vi "Host Image Acquisition Loop.vi"(8 "error in":errorcluster) -> (0 "error out":errorcluster)   [LabVIEW 2013]
doc: "Loop handles the image acquisition communication to FPGA.\nInitialize - Queues up the intialize states\n\nExit"
uses:
  Host Image Acquisition Module Enum.ctl
  Message Passing/MsgQ Loops enum.ctl
  System Status/Status FG Enum.ctl
  File IO/Save Image Module Enum.ctl
  Image Acquisition Settings FG Enum.ctl
  Globals/Simulation Settings Global.vi
  Common/State Machines/State Machine Lib.lvlib
  Message Passing/Main MsgQ.lvlib
panel:
  out "State":string
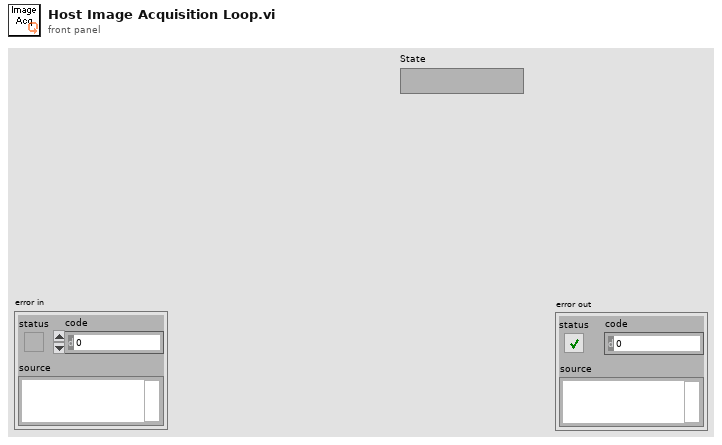
[diagram p1: front panel]
types:
  T1 = typedef "State Machine Lib.lvlib/STATE cluster.ctl" = cluster{"State":string, "Parameters":variant}
  T2 = typedef "Host Image Acquisition Module Enum.ctl" = enum16{"Open FPGA", "Initialize DMA FIFO", "Load Sim Images", "Initialize Acquisition", "Update Sector Parameters", "Start Acquisition", "Aquire Image", "Read Averages", "Cancel Acquisition", "Close FPGA"}
  T3 = typedef "Main MsgQ.lvlib/MsgQ Loops enum.ctl" = enum16{"User Interface", "Image Acq"}
  T4 = typedef "Status FG Enum.ctl" = enum16{"Reset", "Read", "Write"}
  T5 = typedef "Save Image Module Enum.ctl" = enum16{"Create File", "Write to File", "Status", "Close File"}
  T6 = typedef "Image Acquisition Settings FG Enum.ctl" = enum16{"Read", "Write"}
  T7 = typedef "Simulation Settings Cluster.ctl" = cluster{"Sim Enabled?":bool, "Sim Path":path}
  T8 = typedef "Acquisition Settings Cluster.ctl" = cluster{"Image Width":u32, "Image Height":u32, "Frames To Acquire":u32, "Signal Mapping":enum8{"Standard", "Basler 10-tap", "Vosskühler 10-tap"}, "DMA Buffer Size\n(In Images)":u32}
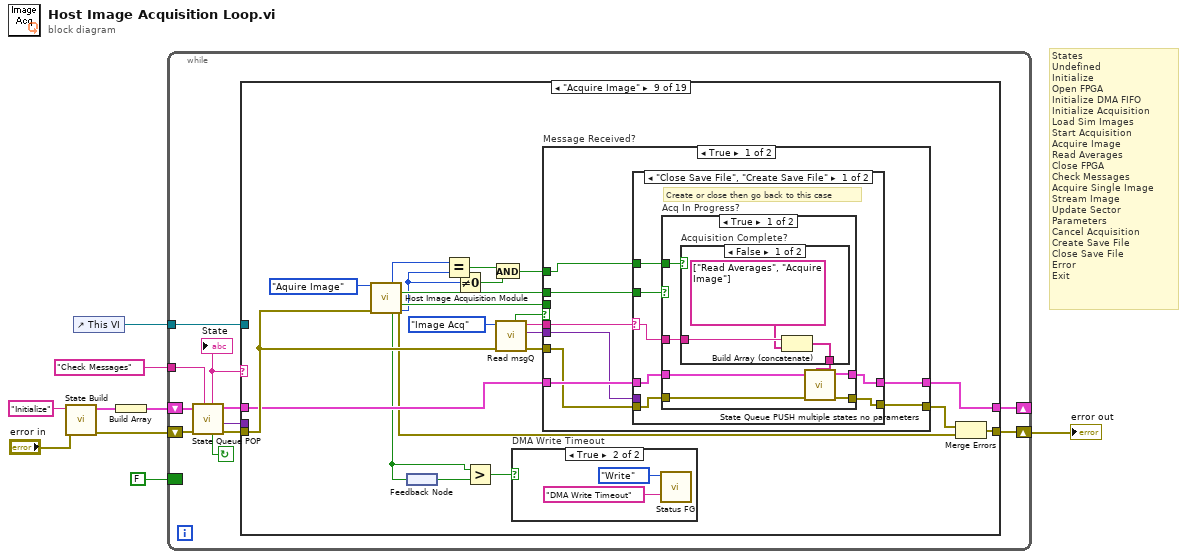
[diagram p0: block diagram]
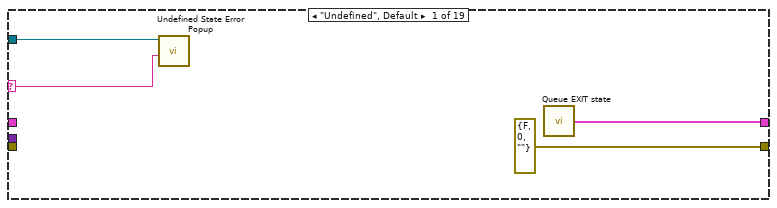
[diagram p2: hidden frame]
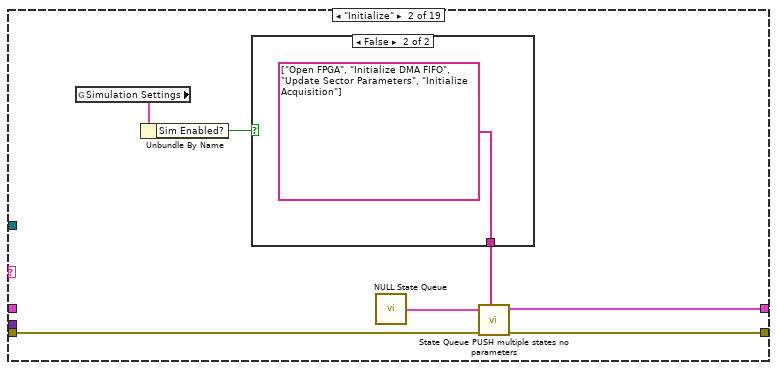
[diagram p3: hidden frame]
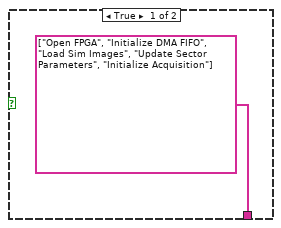
[diagram p4: hidden frame]
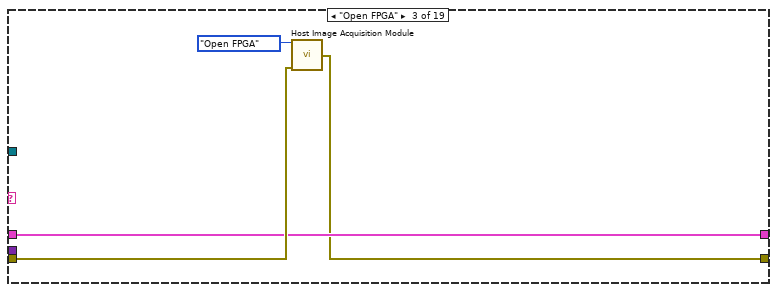
[diagram p5: hidden frame]
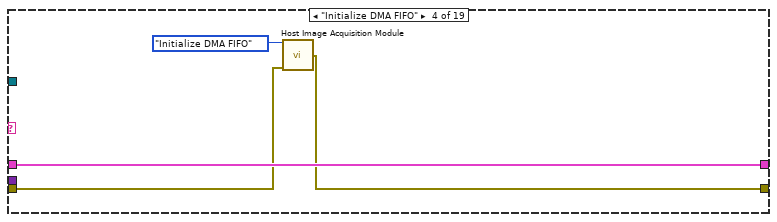
[diagram p6: hidden frame]
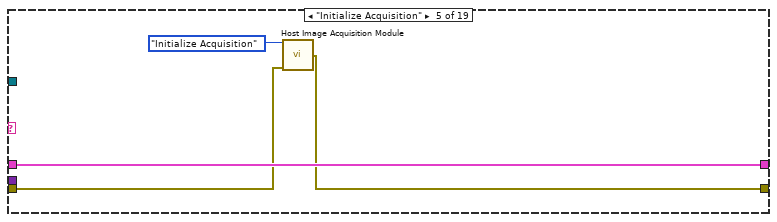
[diagram p7: hidden frame]
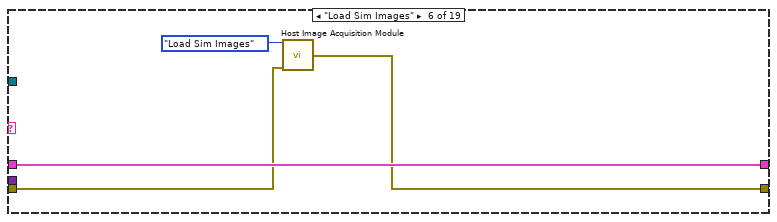
[diagram p8: hidden frame]
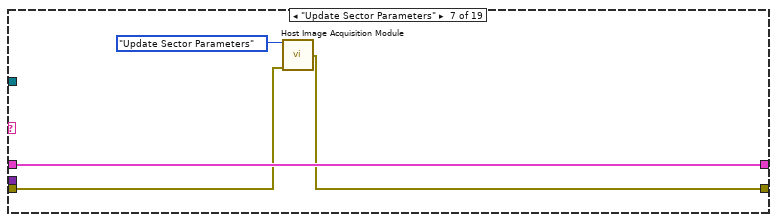
[diagram p9: hidden frame]
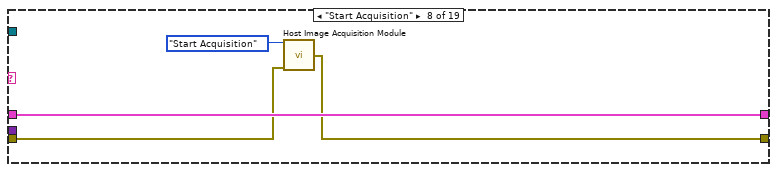
[diagram p10: hidden frame]
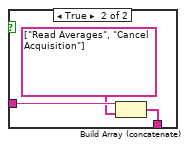
[diagram p12: hidden frame]
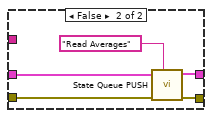
[diagram p13: hidden frame]
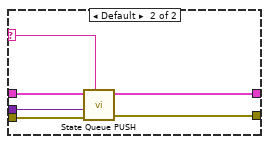
[diagram p14: hidden frame]
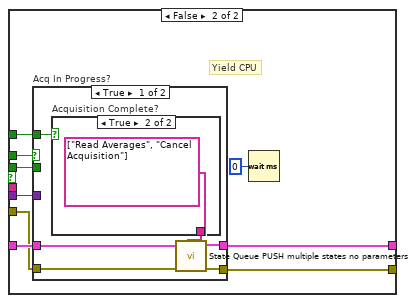
[diagram p15: hidden frame]
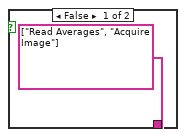
[diagram p16: hidden frame]
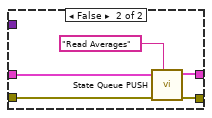
[diagram p17: hidden frame]
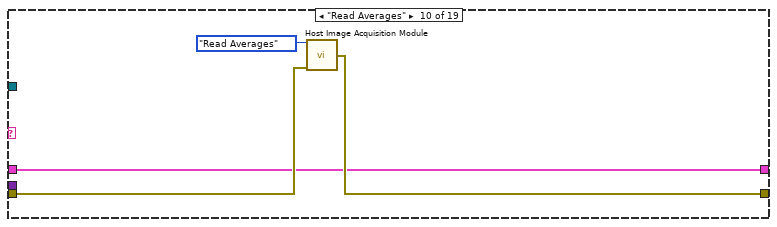
[diagram p18: hidden frame]
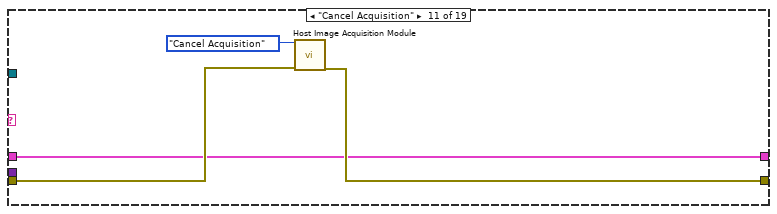
[diagram p19: hidden frame]
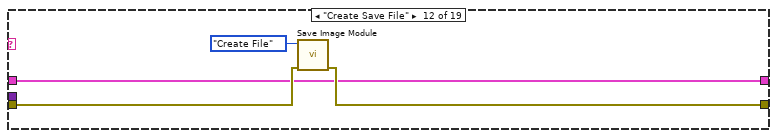
[diagram p20: hidden frame]
diagram:
  # "States\nUndefined\nInitialize\nOpen FPGA\nInitialize DMA FIFO\nInitialize Acquisition\nLoad Sim Images\nStart Acquisition\nAcquire Image\nRead Averages\nClose FPGA\nCheck Messages\nAcquire Single Image\nStream Image\nUpdate Sector Parameters\nCancel Acquisition\nCreate Save File\nClose Save File\nError\nExit"
  n1 = call "State Build.vi"("error in (no error)"="error in", "State"="Initialize") -> ("error out"=w5:errorcluster, "State Out"=w7:T1)  [unwired: 8 in]
  n2 = control-ref of="This VI"() -> (w2:refnum<vi>)
  n3 = Build Array(w7) -> (w6:T1[])
  n4 = while {
    shift-right: [w13] -> _
    shift-left: w6 -> [w20]
    shift-right: [w12] -> w3
    shift-left: w5 -> [w19]
    tunnel: "Check Messages" ("Default state") -> [w17]
    tunnel: w2 -> [w11]
    border: FALSE -> [_]
    stop <- w18 continue-if-true
    n5 = call "State Queue POP.vi"("Default state"=w17, "error in (no error)"=w19, "State que in"=w20) -> ("error out"=w14:errorcluster, "Parameters"=w10:variant, "State que out"=w15:T1[], "Not Exit?"=w18:bool, "State case out"=w16:string)  [unwired: 4 in]
    "State" <- w16
    n6 = case shown="\"Acquire Image\"" w16 {
      selector: w16 -> [w23 _ _ _ _ _ _ _ _ _ _ _ _ _ _ _ _ _ _]
      tunnel: w15 -> [_ _ w35 w41 w45 w49 w53 w57 w77 w143 w147 w151 w157 w162 w169 w184 w205 w225 w232]
      tunnel: w14 -> [_ w31 w36 w40 w44 w48 w52 w56 w78 w145 w149 w153 w155 w161 w171 w191 w195 w228 w231]
      tunnel: [w22 w28 w35 w41 w45 w49 w53 w57 w76 w143 w147 w151 w157 w162 w168 w182 w200 w225 w232] -> w13
      tunnel: [errorcluster {"status"=FALSE, "code"=0, "source"=""} ("error out") w27 w34 w39 w43 w46 w51 w55 w74 w144 w148 w152 w155 w160 w167 w181 w198 w226 w231] -> w12
      tunnel: w11 -> [w24 _ _ _ _ _ _ _ _ _ _ _ _ _ _ _ _ _ _]
      tunnel: w10 -> [_ _ _ _ _ _ _ _ _ _ _ _ _ _ _ _ w204 _ _]
      frame "Undefined", Default {
        n7 = call "Undefined State Error Popup.vi"("String"=w23, "This VI (Caller if unwired)"=w24) -> ()  [unwired: 10 in]
        n8 = call "Queue EXIT state.vi"() -> ("Exit State Q"=w22:T1[])  [unwired: 1 in]
      }
      frame "Initialize" {
        n9 = global read "Simulation Settings Global.vi" "Simulation Settings"() -> (w26:T7)
        n10 = Unbundle By Name(w26) -> ("Sim Enabled?"=w25:bool)
        n11 = case shown="False" w25 {
          tunnel: [string[] ["Open FPGA", "Initialize DMA FIFO", "Load Sim Images", "Update Sector Parameters", "Initialize Acquisition"] ("States to queue") string[] ["Open FPGA", "Initialize DMA FIFO", "Update Sector Parameters", "Initialize Acquisition"] ("States to queue")] -> w29
          frame True {
          }
          frame False {
          }
        }
        n12 = call "NULL State Queue.vi"() -> ("NULL State Queue"=w30:T1[])
        n13 = call "State Queue PUSH multiple states no parameters.vi"("States to queue"=w29, "error in (no error)"=w31, "State que in"=w30) -> ("error out"=w27:errorcluster, "State que out"=w28:T1[])  [unwired: 7 in]
      }
      frame "Open FPGA" {
        n14 = call "Host Image Acquisition Module.vi"("Operation"=Host_Image_Acquisition_Module_Enum."Open FPGA", "error in"=w36) -> ("error out"=w34:errorcluster)  [unwired: 5 in, 8 out]
      }
      frame "Initialize DMA FIFO" {
        n15 = call "Host Image Acquisition Module.vi"("Operation"=Host_Image_Acquisition_Module_Enum."Initialize DMA FIFO", "error in"=w40) -> ("error out"=w39:errorcluster)  [unwired: 5 in, 8 out]
      }
      frame "Initialize Acquisition" {
        n16 = call "Host Image Acquisition Module.vi"("Operation"=Host_Image_Acquisition_Module_Enum."Initialize Acquisition", "error in"=w44) -> ("error out"=w43:errorcluster)  [unwired: 5 in, 8 out]
      }
      frame "Load Sim Images" {
        n17 = call "Host Image Acquisition Module.vi"("Operation"=Host_Image_Acquisition_Module_Enum."Load Sim Images", "error in"=w48) -> ("error out"=w46:errorcluster)  [unwired: 5 in, 8 out]
      }
      frame "Update Sector Parameters" {
        n18 = call "Host Image Acquisition Module.vi"("Operation"=Host_Image_Acquisition_Module_Enum."Update Sector Parameters", "error in"=w52) -> ("error out"=w51:errorcluster)  [unwired: 5 in, 8 out]
      }
      frame "Start Acquisition" {
        n19 = call "Host Image Acquisition Module.vi"("Operation"=Host_Image_Acquisition_Module_Enum."Start Acquisition", "error in"=w56) -> ("error out"=w55:errorcluster)  [unwired: 5 in, 8 out]
      }
      frame "Acquire Image" {
        n20 = call "Host Image Acquisition Module.vi"("Operation"=Host_Image_Acquisition_Module_Enum."Aquire Image", "error in"=w78) -> ("Num Frames read"=w65:u32, "Acq In Progress"=w73:bool, "error out"=w75:errorcluster, "Image Acquired"=w72:bool, "DMA Write Timeout"=w60:bool, "Frames To Acquire"=w61:u32)  [unwired: 5 in, 3 out]
        n21 = feedback-in #1(w60) -> ()
        n22 = feedback #1() -> (w59:bool)
        n23 = Equal?(x=w65, y=w61) -> (x = y?=w64:bool)
        n24 = Not Equal To 0?(x=w61) -> (x != 0?=w62:bool)
        n25 = Greater?(x=w60, y=w59) -> (0:w58:bool)
        n26 = And(x=w64, y=w62) -> (x .and. y?=w63:bool)
        n27 = call "Read msgQ.vi"("error in"=w78, "MsgQ enum"=MsgQ_Loops_enum."Image Acq") -> ("error out"=w68:errorcluster, "Message Received Parameters"=w66:variant, "Message Received String"=w69:string, "Message Recieved?"=w70:bool)  [unwired: 6 in]
        n28 = case "DMA Write Timeout" shown="True" w58 {
          frame False {
          }
          frame True {
            n29 = call "Status FG.vi"("Status In"="DMA Write Timeout", "Operation"=Status_FG_Enum."Write") -> ()  [unwired: 8 in, 2 out]
          }
        }
        n30 = case "Message Received?" shown="True" w70 {
          tunnel: w69 -> [w84 _]
          tunnel: w68 -> [w88 w128]
          tunnel: w77 -> [w89 w129]
          tunnel: [w87 w127] -> w67
          tunnel: [w86 w126] -> w76
          tunnel: w73 -> [w83 w125]
          tunnel: w66 -> [w85 w124]
          tunnel: w72 -> [_ w123]
          tunnel: w63 -> [w82 w122]
          frame True {
            n31 = case shown="\"Close Save File\", \"Create Save File\"" w84 {
              selector: w84 -> [w93 w115]
              tunnel: w89 -> [w95 w120]
              tunnel: w88 -> [w94 w119]
              tunnel: [w90 w118] -> w87
              tunnel: [w91 w117] -> w86
              tunnel: w85 -> [_ w116]
              tunnel: w83 -> [w96 _]
              tunnel: w82 -> [w92 _]
              frame "Close Save File", "Create Save File" {
                # "Create or close then go back to this case"
                n32 = case "Acq In Progress?" shown="True" w96 {
                  tunnel: w95 -> [w103 w114]
                  tunnel: w94 -> [w100 w111]
                  tunnel: [w101 w112] -> w90
                  tunnel: [w102 w113] -> w91
                  tunnel: w92 -> [w98 _]
                  tunnel: w93 -> [w97 _]
                  frame True {
                    n33 = case "Acquisition Complete?" shown="False" w98 {
                      tunnel: [w104 w107] -> w99
                      tunnel: w97 -> [w106 w109]
                      frame False {
                        n34 = Build Array (concatenate)(w106, string[] ["Read Averages", "Acquire Image"] ("States to queue")) -> (w104:string[])
                      }
                      frame True {
                        n35 = Build Array (concatenate)(w109, string[] ["Read Averages", "Cancel Acquisition"] ("States to queue")) -> (w107:string[])
                      }
                    }
                    n36 = call "State Queue PUSH multiple states no parameters.vi"("States to queue"=w99, "error in (no error)"=w100, "State que in"=w103) -> ("error out"=w101:errorcluster, "State que out"=w102:T1[])  [unwired: 7 in]
                  }
                  frame False {
                    n37 = call "State Queue PUSH.vi"("State case"="Read Averages", "error in (no error)"=w111, "State que in"=w114) -> ("error out"=w112:errorcluster, "State que out"=w113:T1[])  [unwired: 7 in]
                  }
                }
              }
              frame Default {
                n38 = call "State Queue PUSH.vi"("State case"=w115, "error in (no error)"=w119, "Parameters"=w116, "State que in"=w120) -> ("error out"=w118:errorcluster, "State que out"=w117:T1[])  [unwired: 6 in]
              }
            }
          }
          frame False {
            # "Yield CPU"
            n39 = case "Acq In Progress?" shown="True" w125 {
              tunnel: w129 -> [w135 w142]
              tunnel: w128 -> [w132 w139]
              tunnel: [w133 w140] -> w127
              tunnel: [w134 w141] -> w126
              tunnel: w124 -> [_ _]
              tunnel: w123 -> [_ _]
              tunnel: w122 -> [w130 _]
              frame True {
                n40 = case "Acquisition Complete?" shown="True" w130 {
                  tunnel: [string[] ["Read Averages", "Acquire Image"] ("States to queue") string[] ["Read Averages", "Cancel Acquisition"] ("States to queue")] -> w131
                  frame False {
                  }
                  frame True {
                  }
                }
                n41 = call "State Queue PUSH multiple states no parameters.vi"("States to queue"=w131, "error in (no error)"=w132, "State que in"=w135) -> ("error out"=w133:errorcluster, "State que out"=w134:T1[])  [unwired: 7 in]
              }
              frame False {
                n42 = call "State Queue PUSH.vi"("State case"="Read Averages", "error in (no error)"=w139, "State que in"=w142) -> ("error out"=w140:errorcluster, "State que out"=w141:T1[])  [unwired: 7 in]
              }
            }
            n43 = Wait (ms)(milliseconds to wait=u32 0) -> ()  [unwired: 1 out]
          }
        }
        n44 = Merge Errors(w67, w75) -> (w74:errorcluster)
      }
      frame "Read Averages" {
        n45 = call "Host Image Acquisition Module.vi"("Operation"=Host_Image_Acquisition_Module_Enum."Read Averages", "error in"=w145) -> ("error out"=w144:errorcluster)  [unwired: 5 in, 8 out]
      }
      frame "Cancel Acquisition" {
        n46 = call "Host Image Acquisition Module.vi"("Operation"=Host_Image_Acquisition_Module_Enum."Cancel Acquisition", "error in"=w149) -> ("error out"=w148:errorcluster)  [unwired: 5 in, 8 out]
      }
      frame "Create Save File" {
        n47 = call "Save Image Module.vi"("error in"=w153, "Mode"=Save_Image_Module_Enum."Create File") -> ("error out"=w152:errorcluster)  [unwired: 8 in, 1 out]
      }
      frame "Close Save File" {
        n48 = call "Save Image Module.vi"("error in"=w155, "Mode"=Save_Image_Module_Enum."Close File") -> ("error out"=w156:errorcluster)  [unwired: 8 in, 1 out]
        n49 = call <vilib>:"Clear Errors.vi"("error in (no error)"=w156) -> ()  [unwired: 6 in, 1 out]
      }
      frame "Close FPGA" {
        n50 = call "Host Image Acquisition Module.vi"("Operation"=Host_Image_Acquisition_Module_Enum."Close FPGA", "error in"=w161) -> ("error out"=w160:errorcluster)  [unwired: 5 in, 8 out]
      }
      frame "Check Messages" {
        n51 = call "Read msgQ.vi"("error in"=w171, "MsgQ enum"=MsgQ_Loops_enum."Image Acq") -> ("error out"=w166:errorcluster, "Message Received Parameters"=w163:variant, "Message Received String"=w165:string, "Message Recieved?"=w170:bool)  [unwired: 6 in]
        n52 = case shown="True" w170 {
          tunnel: w169 -> [w174 w180]
          tunnel: [w174 w179] -> w168
          tunnel: [w173 w178] -> w167
          tunnel: w166 -> [w173 w177]
          tunnel: w165 -> [_ w175]
          tunnel: w163 -> [_ w176]
          frame False {
            # "Yield CPU"
            n53 = Wait (ms)(milliseconds to wait=u32 0) -> ()  [unwired: 1 out]
          }
          frame True {
            n54 = call "State Queue PUSH.vi"("State case"=w175, "error in (no error)"=w177, "Parameters"=w176, "State que in"=w180) -> ("error out"=w178:errorcluster, "State que out"=w179:T1[])  [unwired: 6 in]
          }
        }
      }
      frame "Acquire Single Image" {
        n55 = call "Image Acquisition Settings FG.vi"("error in (no error)"=w191, "Operation"=Image_Acquisition_Settings_FG_Enum."Read") -> ("error out"=w186:errorcluster, "Acquisition Settings Out"=w190:T8)  [unwired: 8 in]
        n56 = Bundle By Name(cluster=w190, "Frames To Acquire"=u32 1) -> (w188:T8)
        n57 = call "Image Acquisition Settings FG.vi"("error in (no error)"=w186, "Acquisition Settings In"=w188, "Operation"=Image_Acquisition_Settings_FG_Enum."Write") -> ("error out"=w185:errorcluster)  [unwired: 7 in, 1 out]
        n58 = call "State Queue PUSH multiple states no parameters.vi"("States to queue"=string[] ["Start Acquisition", "Acquire Image"], "error in (no error)"=w185, "State que in"=w184) -> ("error out"=w181:errorcluster, "State que out"=w182:T1[])  [unwired: 7 in]
      }
      frame "Stream Image" {
        n59 = global read "Simulation Settings Global.vi" "Simulation Settings"() -> (w196:T7)
        n60 = Unbundle By Name(w196) -> ("Sim Enabled?"=w193:bool)
        n61 = Variant To Data(error in=w195, type=TRUE, Variant=w204) -> (data=w202:bool, error out=w194:errorcluster)
        n62 = case "Enable Stream?" shown="True" w202 {
          tunnel: w194 -> [w206 w213]
          tunnel: w205 -> [w207 w212]
          tunnel: [w207 w212] -> w201
          tunnel: [w206 w211] -> w199
          tunnel: [string[] ["Cancel Acquisition", "Close Save File"] ("States to queue") string[] ["Start Acquisition", "Acquire Image"] ("States to queue")] -> w197
          tunnel: w193 -> [_ w209]
          frame False {
          }
          frame True {
            n63 = case shown="False" w209 {
              tunnel: w213 -> [w220 w222]
              tunnel: [w214 w222] -> w211
              frame False {
                n64 = call "Image Acquisition Settings FG.vi"("error in (no error)"=w220, "Operation"=Image_Acquisition_Settings_FG_Enum."Read") -> ("error out"=w215:errorcluster, "Acquisition Settings Out"=w219:T8)  [unwired: 8 in]
                n65 = Bundle By Name(cluster=w219, "Frames To Acquire"=u32 0) -> (w217:T8)
                n66 = call "Image Acquisition Settings FG.vi"("error in (no error)"=w215, "Acquisition Settings In"=w217, "Operation"=Image_Acquisition_Settings_FG_Enum."Write") -> ("error out"=w214:errorcluster)  [unwired: 7 in, 1 out]
              }
              frame True {
              }
            }
          }
        }
        n67 = call "State Queue PUSH multiple states no parameters.vi"("States to queue"=w197, "error in (no error)"=w199, "State que in"=w201) -> ("error out"=w198:errorcluster, "State que out"=w200:T1[])  [unwired: 7 in]
      }
      frame "Error" {
        n68 = Unbundle By Name(w228) -> ("source"=w229:string)
        n69 = Concatenate Strings("Error: " ("string"), w229) -> (w224:string)
        n70 = call "Status FG.vi"("Status In"=w224, "Operation"=Status_FG_Enum."Write") -> ()  [unwired: 8 in, 2 out]
        n71 = call "Broadcast Exit.vi"("error in"=errorcluster {"status"=FALSE, "code"=0, "source"=""}) -> ("error out"=w226:errorcluster)  [unwired: 10 in]
      }
      frame "Exit" {
      }
    }
  }
  "error out" <- w3
